vi "is dictionary empty.vi"(11 "data dictionary in":refnum<class "data bus dictionary.lvclass">) -> (2 "empty?":bool, 3 "data dictionary out":refnum<class "data bus dictionary.lvclass">)   [LabVIEW 2013, in "data bus dictionary.lvclass"]
doc: "Determines whether or not a dictionary is empty."
uses:
  data bus dictionary.lvclass
  data bus dictionary.lvclass/data bus dictionary.ctl
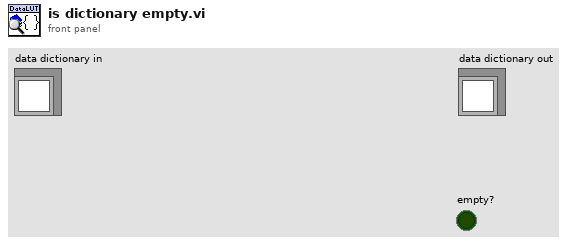
[diagram p1: front panel]
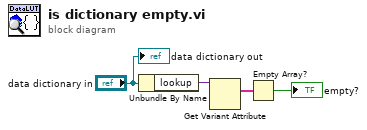
[diagram p0: block diagram]
diagram:
  n1 = Unbundle By Name("data dictionary in") -> ("lookup"=w3:variant)
  n2 = Get Variant Attribute(Variant=w3) -> (names=w2:string[])  [unwired: 3 in, 3 out]
  n3 = Empty Array?(array=w2) -> (empty?=→"empty?":bool)
  "data dictionary out" <- "data dictionary in"
